vi "calcLatInc.vi"(1 "FOV (mm)":dbl=0.53248, 2 "% FOV overlap":i32=10) -> (0 "Lateral increment (mm)":dbl=0.479232)   [LabVIEW 2015]
panel:
  out "FOV (mm)":dbl=0.53248
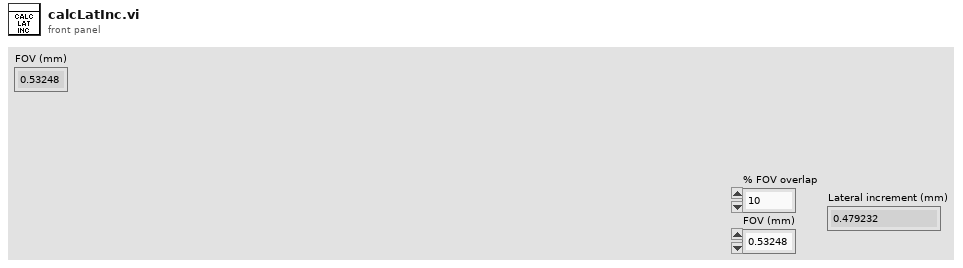
[diagram p1: front panel]
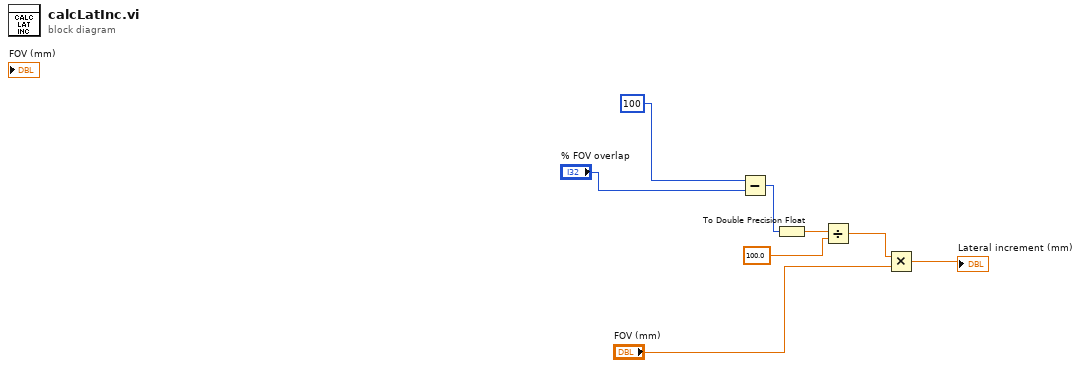
[diagram p0: block diagram]
diagram:
  n1 = Subtract(x=100 ("y"), y="% FOV overlap") -> (x-y=w5:i32)
  n2 = To Double Precision Float(number=w5) -> (double precision float=w6:dbl)
  n3 = Divide(x=w6, y=100.0) -> (x/y=w8:dbl)
  n4 = Multiply(x=w8, y="FOV (mm)") -> (x*y=→"Lateral increment (mm)":dbl)
